vi "XML操作.vi"(7 "File Name":string, 8 "SAVE/READ":bool, 9 "Save":variant, 10 "Read":variant, 11 "ProgramNO.":i32) -> (3 "数组":variant[](array[variant]))   [LabVIEW 2014]
uses:
  <vilib>/Utility/xml.llb/Write to XML File(string).vi
  <vilib>/Utility/xml.llb/Read From XML File(array).vi
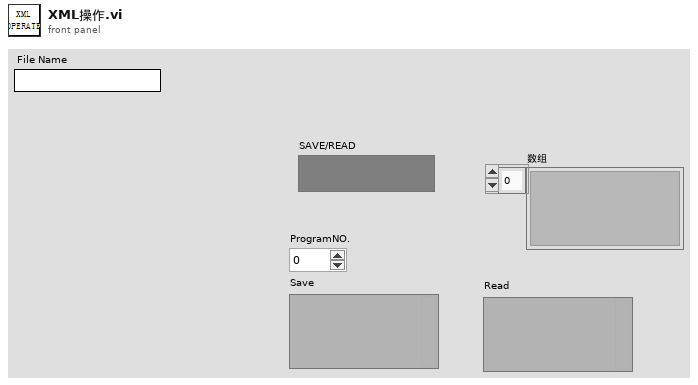
[diagram p1: front panel]
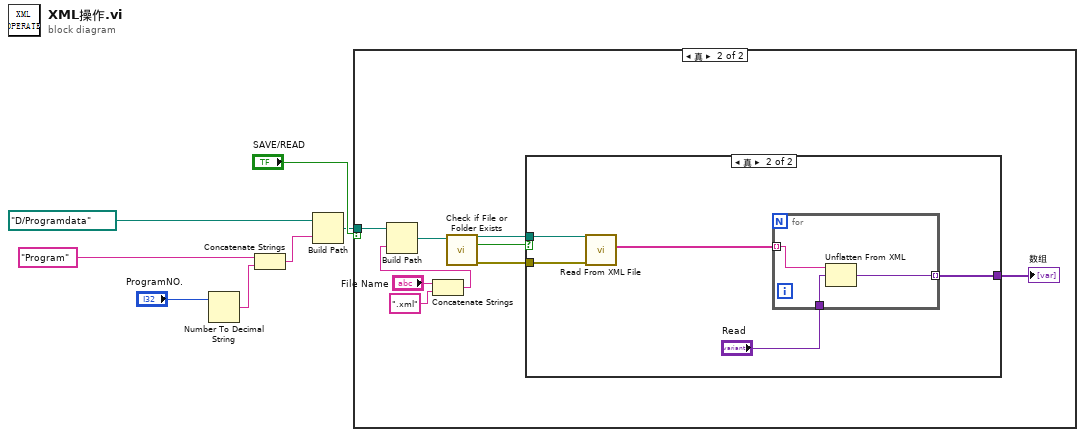
[diagram p0: block diagram]
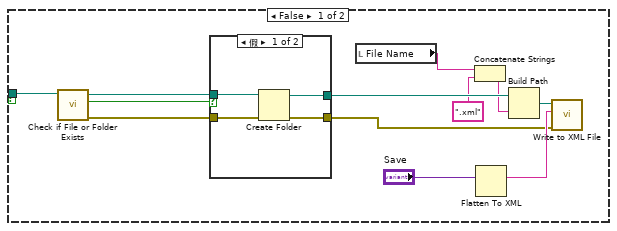
[diagram p2: hidden frame]
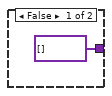
[diagram p4: hidden frame]
diagram:
  n1 = Number To Decimal String(number="ProgramNO.") -> (decimal integer string=w6:string)  [unwired: 1 in]
  n2 = Concatenate Strings("Program" ("名称或相对路径"), w6) -> (w7:string)
  n3 = Build Path(base path=path "D:/Programdata" ("基路径"), name or relative path=w7) -> (appended path=w3:path)
  n4 = case shown="真" "SAVE/READ" {
    tunnel: w3 -> [w19 w30]
    frame False {
      n5 = call <vilib>:"Check if File or Folder Exists.vi"("path"=w19) -> ("error out"=w17:errorcluster, "file or folder exists?"=w16:bool, "dup path"=w18:path)  [unwired: 8 in]
      n6 = case shown="假" w16 {
        tunnel: [w21 w25] -> w13
        tunnel: w18 -> [w23 w25]
        tunnel: [w20 w24] -> w12
        tunnel: w17 -> [w22 w24]
        frame False {
          n7 = Create Folder(path (use dialog)=w23, error in=w22) -> (created path=w21:path, error out=w20:errorcluster)  [unwired: 1 in, 1 out]
        }
        frame True {
        }
      }
      n8 = local read "File Name"() -> (w10:string)
      n9 = Concatenate Strings(w10, ".xml" ("名称或相对路径")) -> (w8:string)
      n10 = Flatten To XML(anything="Save") -> (xml string=w15:string)
      n11 = Build Path(base path=w13, name or relative path=w8) -> (appended path=w14:path)
      n12 = call-poly <vilib>:"Write to XML File.vi"("error in (no error)"=w12, "XML Input"=w15, "XML File Path"=w14) -> ()  [unwired: 6 in, 3 out]
    }
    frame True {
      n13 = Concatenate Strings("File Name", ".xml" ("名称或相对路径")) -> (w26:string)
      n14 = Build Path(base path=w30, name or relative path=w26) -> (appended path=w32:path)
      n15 = call <vilib>:"Check if File or Folder Exists.vi"("path"=w32) -> ("error out"=w33:errorcluster, "file or folder exists?"=w29:bool, "dup path"=w34:path)  [unwired: 8 in]
      n16 = case shown="真" w29 {
        tunnel: w34 -> [_ w40]
        tunnel: w33 -> [_ w39]
        tunnel: [variant[] [] w37] -> w31
        frame False {
        }
        frame True {
          n17 = call-poly <vilib>:"Read From XML File.vi"("error in (no error)"=w39, "XML File Path"=w40) -> ("XML Elements"=w36:string[])  [unwired: 7 in, 2 out]
          n18 = for {
            tunnel: "Read" -> [w43]
            tunnel: [w42] -> w37 mode=indexing
            tunnel: w36 -> [w41] mode=indexing
            n19 = Unflatten From XML(xml string=w41, type=w43) -> (value=w42:variant)  [unwired: 1 in, 1 out]
          }
        }
      }
      "数组" <- w31
    }
  }
